vi "Read Annotation Ground Truth.vi"(8 "Error In":errorcluster, 9 "Filename without extension":string, 10 "Folder":path, 11 "Total no frames playback":i32) -> (0 "Error Out":errorcluster, 1 "annotation file path":path, 2 "Annotation List":T1[](array[typedef]) {"Frame Start" min=0}, 3 "Annotation array (strings)":string[](array[string]), 4 "annotation list exists?":bool)   [LabVIEW 2017]
uses:
  Controls/Annotation Sequence Details.ctl
  <vilib>/Utility/file.llb/Read Delimited Spreadsheet (string).vi
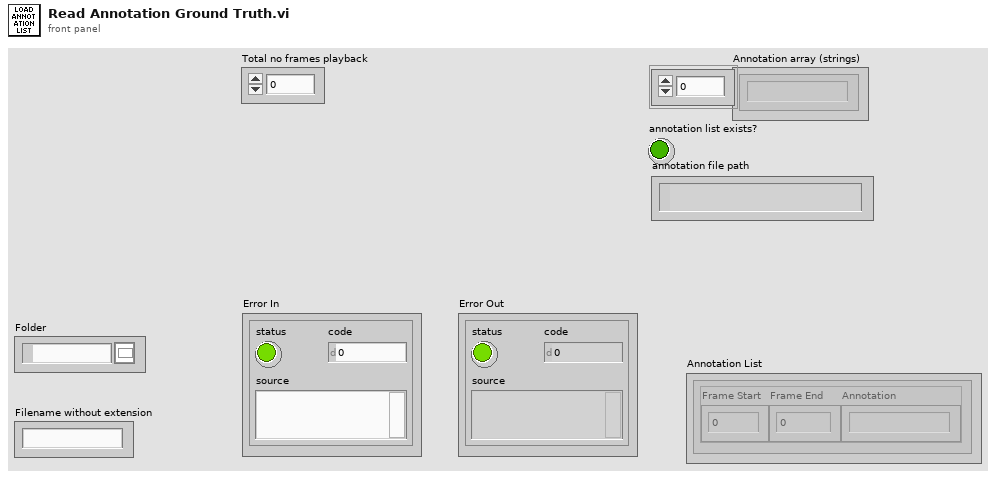
[diagram p1: front panel]
types:
  T1 = typedef "Annotation Sequence Details.ctl" = cluster{"Frame Start":i32, "Frame End":i32, "Annotation":string}
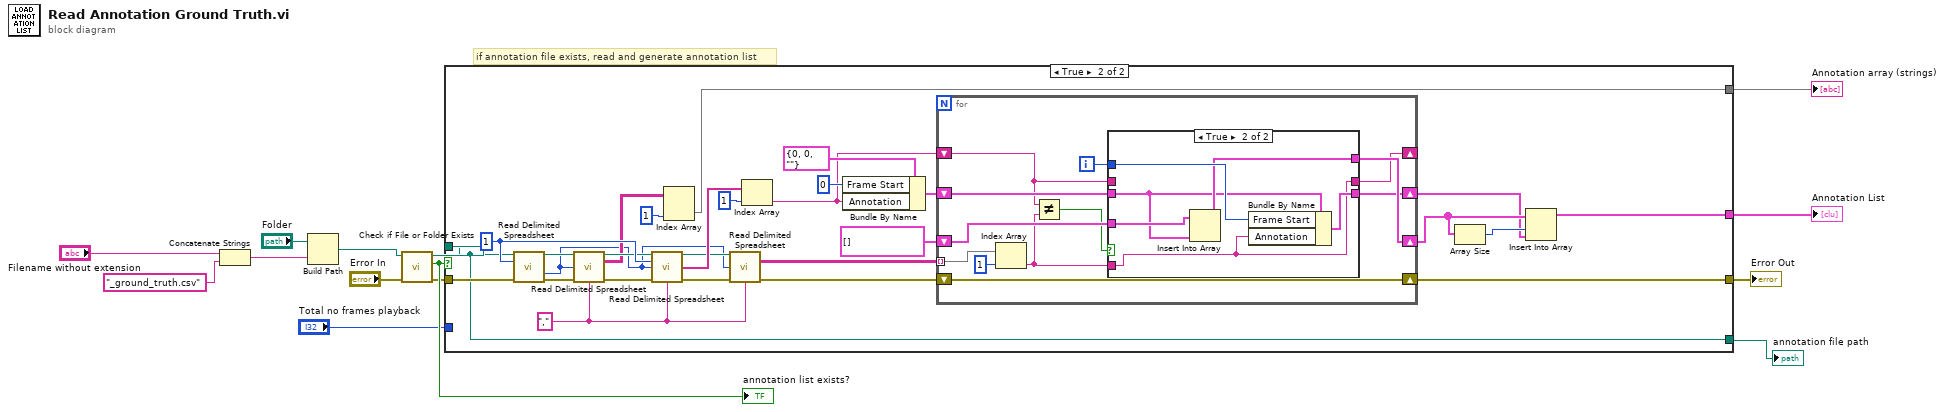
[diagram p0: block diagram]
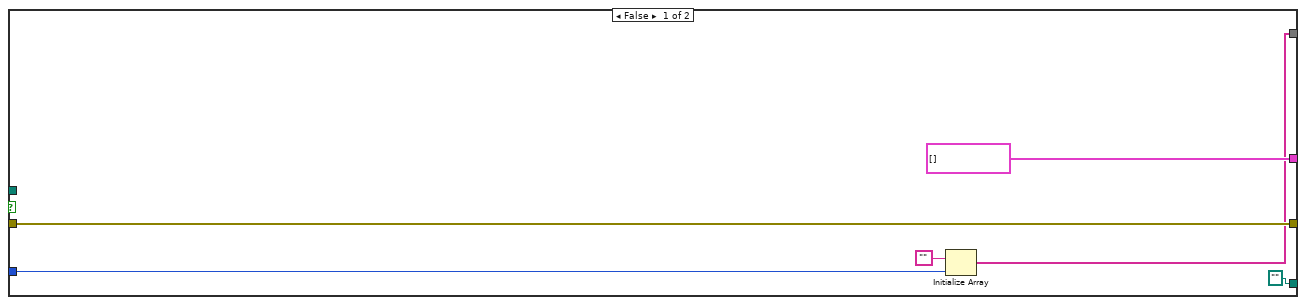
[diagram p2: hidden frame]
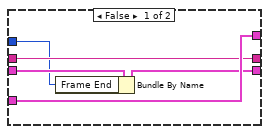
[diagram p3: hidden frame]
diagram:
  # "if annotation file exists, read and generate annotation list"
  n1 = Concatenate Strings("Filename without extension", "_ground_truth.csv" ("string")) -> (w11:string)
  n2 = Build Path(base path="Folder", name or relative path=w11) -> (appended path=w10:path)
  n3 = call <vilib>:"Check if File or Folder Exists.vi"("error in (no error)"="Error In", "path"=w10) -> ("error out"=w6:errorcluster, "file or folder exists?"=w8:bool, "dup path"=w4:path)  [unwired: 7 in]
  "annotation list exists?" <- w8
  n4 = case shown="True" w8 {
    tunnel: [T1[] [] ("Annotation List") w24] -> w7
    tunnel: w6 -> [w19 w48]
    tunnel: [w19 w35] -> w5
    tunnel: w4 -> [_ w25]
    tunnel: [w17 w27] -> w3
    tunnel: "Total no frames playback" -> [w16 _]
    tunnel: [path "" w25] -> w1
    frame False {
      n5 = Initialize Array("", w16) -> (w17:string[])
    }
    frame True {
      w30 = "," ("delimiter (\\t)")
      w42 = 1 ("number of rows (all:-1)")
      n6 = call-poly <vilib>:"Read Delimited Spreadsheet.vi"("file path (dialog if empty)"=w25, "number of rows (all:-1)"=w42, "error in (no error)"=w48) -> ("new file path (Not A Path if cancelled)"=w32:path, "mark after read (chars.)"=w26:i32, "error out"=w34:errorcluster)  [unwired: 7 in, 3 out]
      n7 = call-poly <vilib>:"Read Delimited Spreadsheet.vi"("file path (dialog if empty)"=w32, "start of read offset (chars.:0)"=w26, "error in (no error)"=w34, "delimiter (\\t)"=w30) -> ("new file path (Not A Path if cancelled)"=w31:path, "all rows"=w29:string[][], "error out"=w33:errorcluster)  [unwired: 6 in, 3 out]
      n8 = call-poly <vilib>:"Read Delimited Spreadsheet.vi"("file path (dialog if empty)"=w31, "number of rows (all:-1)"=w42, "start of read offset (chars.:0)"=w26, "error in (no error)"=w33, "delimiter (\\t)"=w30) -> ("new file path (Not A Path if cancelled)"=w36:path, "first row"=w40:string[], "error out"=w45:errorcluster)  [unwired: 5 in, 3 out]
      n9 = Index Array(array=w29, index (col)=1 ("disabled index (col)")) -> (element=w27:string[])  [unwired: 1 in]
      n10 = call-poly <vilib>:"Read Delimited Spreadsheet.vi"("file path (dialog if empty)"=w36, "start of read offset (chars.:0)"=w26, "error in (no error)"=w45, "delimiter (\\t)"=w30) -> ("all rows"=w43:string[][], "error out"=w44:errorcluster)  [unwired: 6 in, 4 out]
      n11 = Index Array(array=w40, index=1) -> (element=w37:string)
      n12 = Bundle By Name(cluster=T1 {"Frame Start"=0, "Frame End"=0, "Annotation"=""} ("Annotation Sequence Details"), "Frame Start"=0, "Annotation"=w37) -> (w39:T1)
      n13 = for {
        tunnel: w43 -> [w57] mode=indexing
        shift-right: [w60] -> w23
        shift-left: T1[] [] ("Annotation List") -> [w59]
        shift-right: [w51] -> _
        shift-left: w37 -> [w50]
        shift-right: [w54] -> w35
        shift-left: w44 -> [w54]
        shift-right: [w55] -> w21
        shift-left: w39 -> [w58]
        i -> [w49]
        n14 = Index Array(array=w57, index=1) -> (element=w52:string)
        n15 = Not Equal?(x=w50, y=w52) -> (x != y?=w53:bool)
        n16 = case shown="True" w53 {
          tunnel: [w65 w68] -> w60
          tunnel: w59 -> [w65 w67]
          tunnel: w58 -> [w63 w66]
          tunnel: [w62 w70] -> w55
          tunnel: w49 -> [w61 w71]
          tunnel: w52 -> [_ w69]
          tunnel: [w64 w69] -> w51
          tunnel: w50 -> [w64 _]
          frame False {
            n17 = Bundle By Name(cluster=w63, "Frame End"=w61) -> (w62:T1)
          }
          frame True {
            n18 = Insert Into Array(array=w67, new element=w66) -> (w68:T1[])  [unwired: 1 in]
            n19 = Bundle By Name(cluster=w66, "Frame Start"=w71, "Annotation"=w69) -> (w70:T1)
          }
        }
      }
      n20 = Array Size(array=w23) -> (size(s)=w22:i32)
      n21 = Insert Into Array(array=w23, index=w22, new element=w21) -> (w24:T1[])
    }
  }
  "Error Out" <- w5
  "Annotation List" <- w7
  "Annotation array (strings)" <- w3
  "annotation file path" <- w1
